vi "Write Execution Time.vi"(8 "error in (no error)":errorcluster, 10 "values in":dbl[](array[numeric]), 11 "execution unit":refnum<class "Execution Unit.lvclass">) -> (0 "error out":errorcluster, 2 "values out":dbl[](array[numeric]), 3 "execution unit out":refnum<class "Execution Unit.lvclass">)   [LabVIEW 2020, in "AIM MIL-STD-1553 Engine.lvlib" / "Implementation.lvlib" / "Execution Unit.lvclass"]
uses:
  Execution Unit.lvclass
  Execution Unit.lvclass/Execution Unit.ctl
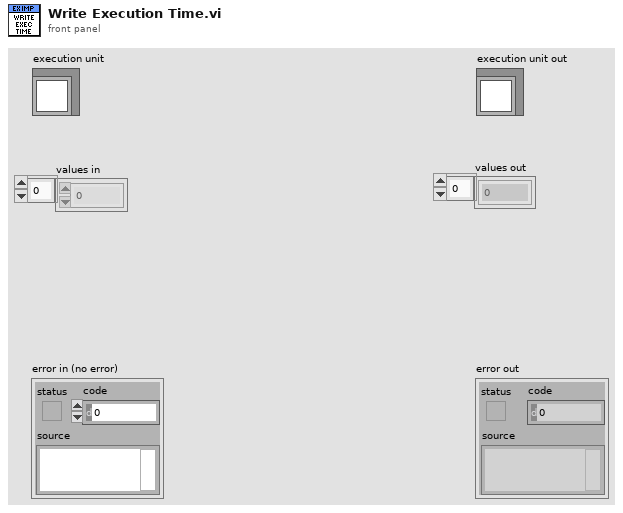
[diagram p1: front panel]
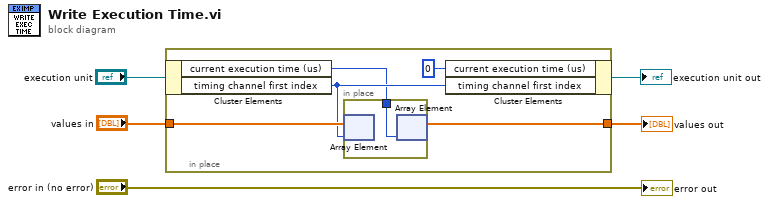
[diagram p0: block diagram]
diagram:
  n1 = in-place {
    in-place-border: "values in" -> [w9]
    in-place-border: [w6] -> w3
    n2 = in-place-cluster #1("execution unit") -> ("current execution time (us)"=w7:i32, "timing channel first index"=w8:i32)
    n3 = in-place {
      in-place-border: w7 -> [w11]
      n4 = in-place-array #2(w9, w8) -> ()  [unwired: 1 out]
      n5 = in-place-array #2(w11) -> (w6:dbl[])  [unwired: 1 out]
    }
    n6 = in-place-cluster #1("current execution time (us)"=0, "timing channel first index"=w8) -> (→"execution unit out":refnum<class "Execution Unit.lvclass">)
  }
  "values out" <- w3
  "error out" <- "error in (no error)"
